vi "UDP Write String Test.vi"() -> ()   [LabVIEW 2014, in "ESP8266 WiFi Wrapper.lvlib"]
uses:
  <vilib>/Aledyne-TSXperts/Arduino Compatible Compiler for LabVIEW/addons/ESP8266 WiFi Wrapper/ESP8266 WiFi Wrapper.lvlib
panel:
  out "Chars written":u8
  out "Successful end packet?":bool
  out "Successful start packet?":bool
  out "Error Out":errorcluster
  in  "Error In":errorcluster
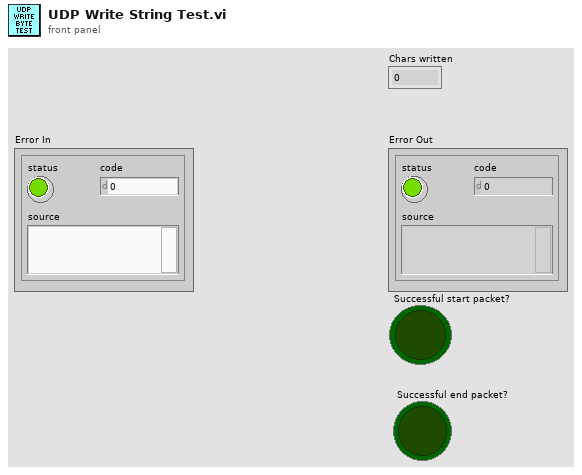
[diagram p1: front panel]
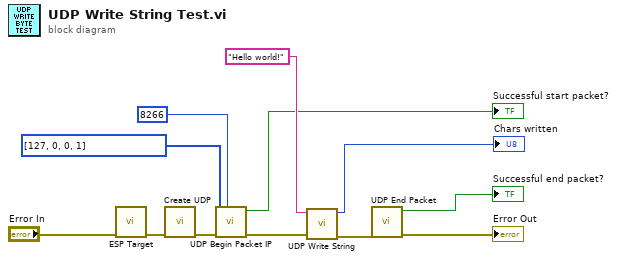
[diagram p0: block diagram]
diagram:
  n1 = call <vilib>:"ESP Target.vi"("Error In"="Error In") -> ("Error Out"=w11:errorcluster)  [unwired: 10 in]
  n2 = call <vilib>:"Create UDP.vi"("Error In"=w11) -> ("Error Out"=w1:errorcluster)  [unwired: 10 in]
  n3 = call <vilib>:"UDP Begin Packet IP.vi"("Port"=i16 8266, "Error In"=w1, "IP Address"=u8[] [127, 0, 0, 1]) -> ("Error Out"=w2:errorcluster, "Successful?"=→"Successful start packet?":bool)  [unwired: 7 in]
  n4 = call <vilib>:"UDP Write String.vi"("Error In"=w2, "String to write"="Hello world!") -> ("Error Out"=w8:errorcluster, "Chars written"=→"Chars written":u8)  [unwired: 8 in]
  n5 = call <vilib>:"UDP End Packet.vi"("Error In"=w8) -> ("Error Out"=→"Error Out":errorcluster, "Successful?"=→"Successful end packet?":bool)  [unwired: 9 in]
